vi "Acquire.vi"(8 "error in (no error)":errorcluster, 11 "DAQmxDI in":refnum<class "DAQmxDI.lvclass">) -> (0 "error out":errorcluster, 3 "DAQmxDI out":refnum<class "DAQmxDI.lvclass">)   [LabVIEW 2023, in "VolatusDAQ.lvlib" / "DAQmxDI.lvclass"]
uses:
  DAQmxDI.lvclass
  DAQmxDI.lvclass/DAQmxDI.ctl
  Volatus/MessageQ/MessageQ.lvclass/MessageQ.ctl
  <vilib>/DAQmx/read.llb/DAQmx Read (Digital 2D U32 NChan NSamp).vi
  <vilib>/DAQmx/read.llb/DAQmx Read (Digital 1D U32 NChan 1Samp).vi
  Volatus/MessageQ/Send.vi
  <vilib>/DAQmx/miscellaneous.llb/DAQmx Fill In Error Info.vi
  VolatusData/VolatusData.lvlib
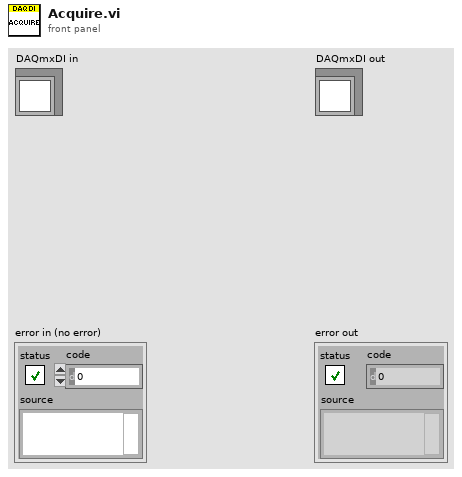
[diagram p1: front panel]
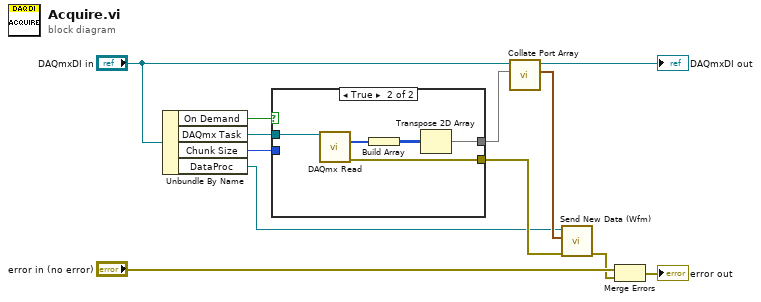
[diagram p0: block diagram]
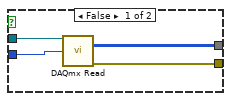
[diagram p2: hidden frame]
diagram:
  n1 = Unbundle By Name("DAQmxDI in") -> ("On Demand"=w1:bool, "DAQmx Task"=w10:refnum<k21>, "Chunk Size"=w2:i32, "DataProc"=w3:refnum<class "MessageQ.lvclass">)
  n2 = case shown="True" w1 {
    tunnel: [w16 w19] -> w12
    tunnel: w10 -> [w15 w21]
    tunnel: [w14 w17] -> w4
    tunnel: w2 -> [w13 _]
    frame False {
      n3 = call-poly <vilib>:"DAQmx Read.vi"("task/channels in"=w15, "number of samples per channel"=w13) -> ("data"=w14:u32[][], "error out"=w16:errorcluster)  [unwired: 11 in, 1 out]
    }
    frame True {
      n4 = call-poly <vilib>:"DAQmx Read.vi"("task/channels in"=w21) -> ("data"=w20:u32[], "error out"=w19:errorcluster)  [unwired: 12 in, 1 out]
      n5 = Build Array(w20) -> (w18:u32[][])
      n6 = Transpose 2D Array(2D array=w18) -> (transposed array=w17:u32[][])
    }
  }
  n7 = call "Collate Port Array.vi"("data"=w4, "DAQmxDI in"="DAQmxDI in") -> ("Waveforms"=w5:waveform(dbl)[], "DAQmxDI out"=→"DAQmxDI out":refnum<class "DAQmxDI.lvclass">)  [unwired: 7 in, 1 out]
  n8 = call "Send New Data (Wfm).vi"("error in (no error)"=w12, "Channels"=w5, "MessageQ"=w3) -> ("error out"=w8:errorcluster)  [unwired: 8 in]
  n9 = Merge Errors("error in (no error)", w8) -> (→"error out":errorcluster)
